vi "S-Curve Newton Method Velocity.vi"(4 "v_f":dbl, 6 "v_i":dbl, 7 "err":dbl, 8 "g":dbl, 9 "j":dbl, 10 "a":dbl, 11 "t":dbl) -> (3 "v_out":dbl)   [LabVIEW 2025]
uses:
  <vilib>/ptbypt/NI_PtbyPt.lvlib
panel:
  out "iterations":i32
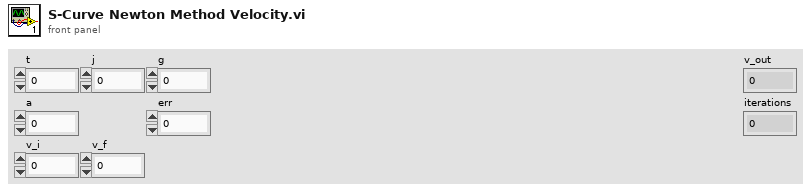
[diagram p1: front panel]
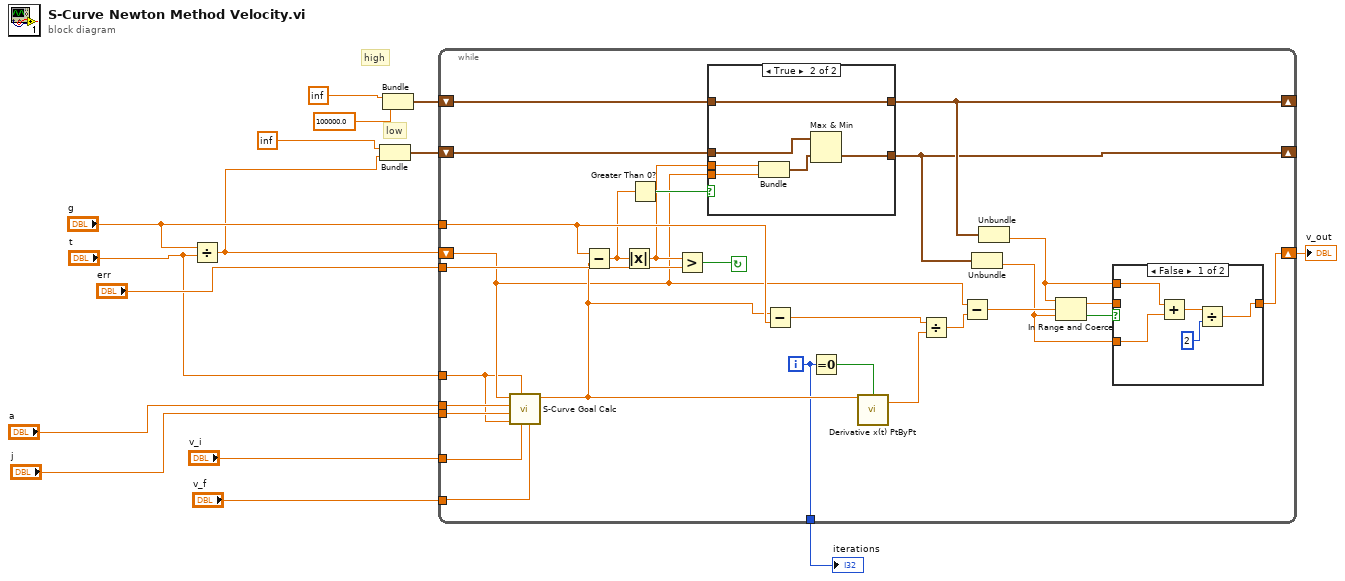
[diagram p0: block diagram]
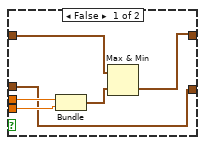
[diagram p2: hidden frame]
diagram:
  # "low"
  # "high"
  n1 = Divide(x="g", y="t") -> (x/y=w4:dbl)
  n2 = Bundle(inf, w4) -> (w7:cluster{dbl, dbl})  [unwired: 1 in]
  n3 = Bundle(inf, 100000.0) -> (w2:cluster{dbl, dbl})  [unwired: 1 in]
  n4 = while {
    tunnel: "a" -> [w43]
    tunnel: "j" -> [w42]
    tunnel: "v_i" -> [w41]
    tunnel: "v_f" -> [w40]
    shift-right: [w20] -> w10
    shift-left: w4 -> [w17]
    tunnel: "g" -> [w36]
    tunnel: "err" -> [w39]
    shift-right: [w25] -> _
    shift-left: w2 -> [w26]
    shift-right: [w24] -> _
    shift-left: w7 -> [w28]
    tunnel: [w23] -> w6
    tunnel: "t" -> [w16]
    i -> [w23]
    stop <- w38 continue-if-true
    n5 = call "S-Curve Goal Calc.vi"("v_f"=w40, "v_i"=w41, "x"=w16, "t"=w16, "j"=w42, "a"=w43, "v"=w17) -> ("goal"=w33:dbl)  [unwired: 4 in]
    n6 = Subtract(x=w36, y=w33) -> (x-y=w30:dbl)
    n7 = Absolute Value(x=w30) -> (abs(x)=w27:dbl)
    n8 = Greater Than 0?(x=w30) -> (x > 0?=w29:bool)
    n9 = Greater?(x=w27, y=w39) -> (0:w38:bool)
    n10 = case shown="True" w29 {
      tunnel: w28 -> [w44 w52]
      tunnel: w27 -> [w48 w55]
      tunnel: w17 -> [w47 w54]
      tunnel: [w44 w51] -> w24
      tunnel: w26 -> [w46 w50]
      tunnel: [w45 w50] -> w25
      frame False {
        n11 = Bundle(w48, w47) -> (w49:cluster{dbl, dbl})  [unwired: 1 in]
        n12 = Max & Min(x=w46, y=w49) -> (min(x,y)=w45:cluster{dbl, dbl})  [unwired: 1 out]
      }
      frame True {
        n13 = Bundle(w55, w54) -> (w53:cluster{dbl, dbl})  [unwired: 1 in]
        n14 = Max & Min(x=w52, y=w53) -> (min(x,y)=w51:cluster{dbl, dbl})  [unwired: 1 out]
      }
    }
    n15 = Subtract(x=w33, y=w36) -> (x-y=w35:dbl)
    n16 = Equal To 0?(x=w23) -> (x = 0?=w31:bool)
    n17 = call <vilib>:"Derivative x(t) PtByPt.vi"("initialize"=w31, "x"=w33) -> ("dx/dt"=w32:dbl)  [unwired: 2 in, 1 out]
    n18 = Divide(x=w35, y=w32) -> (x/y=w37:dbl)
    n19 = Subtract(x=w17, y=w37) -> (x-y=w34:dbl)
    n20 = Unbundle(w24) -> (w18:dbl)  [unwired: 1 out]
    n21 = Unbundle(w25) -> (w19:dbl)  [unwired: 1 out]
    n22 = In Range and Coerce(upper limit=w19, x=w34, lower limit=w18) -> (coerced(x)=w21:dbl, In Range?=w22:bool)
    n23 = case shown="False" w22 {
      tunnel: w21 -> [_ w61]
      tunnel: [w56 w61] -> w20
      tunnel: w19 -> [w60 _]
      tunnel: w18 -> [w59 _]
      frame False {
        n24 = Add(x=w60, y=w59) -> (x+y=w58:dbl)
        n25 = Divide(x=w58, y=2) -> (x/y=w56:dbl)
      }
      frame True {
      }
    }
  }
  "v_out" <- w10
  "iterations" <- w6
